vi "virtual_temp_continously.vi"() -> ()   [LabVIEW 2019]
panel:
  out "Waveform Chart":dynamicdata(graph)
  in  "stop (F)":bool
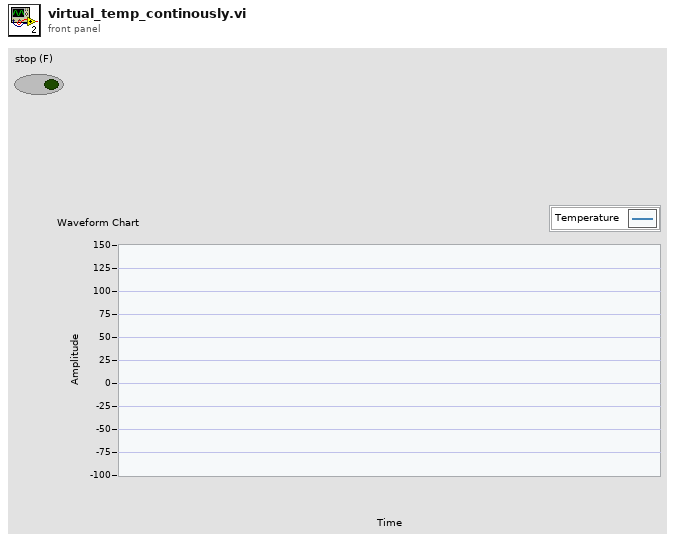
[diagram p1: front panel]
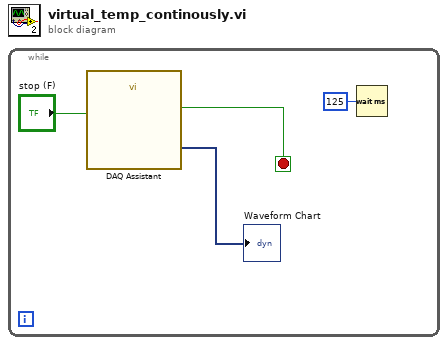
[diagram p0: block diagram]
diagram:
  n1 = while {
    stop <- w3 stop-if-true
    n2 = call "DAQ Assistant"("stop (F)"="stop (F)") -> ("data"=→"Waveform Chart":dynamicdata, "stopped"=w3:bool)  [unwired: 15 in, 2 out]
    n3 = Wait (ms)(milliseconds to wait=u32 125) -> ()  [unwired: 1 out]
  }
